vi "ANdroid_info_pusher.vi"(10 "IndexerIn":i32) -> (2 "indexout":i32, 3 "spreadsheet string":string)   [LabVIEW 2015]
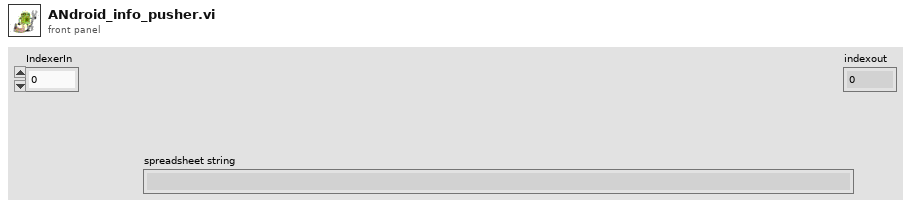
[diagram p1: front panel]
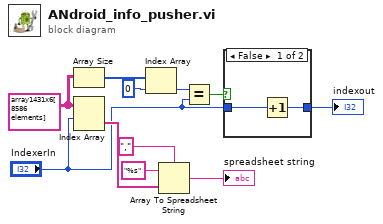
[diagram p0: block diagram]
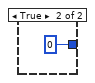
[diagram p2: hidden frame]
diagram:
  w2 = string[][] array1431x6[8586 elements] ("subarray 2")
  n1 = Array Size(array=w2) -> (size(s)=w7:i32[])
  n2 = Index Array(array=w2, index (row)="IndexerIn") -> (element=w9:string[])  [unwired: 1 in]
  n3 = Index Array(array=w7, index=0) -> (element=w5:i32)
  n4 = Array To Spreadsheet String(delimiter (Tab)=",", array=w9, 3:"%s" ("format string")) -> (spreadsheet string=→"spreadsheet string":string)
  n5 = Equal?(x=w5, y="IndexerIn") -> (x = y?=w4:bool)
  n6 = case shown="False" w4 {
    tunnel: [w13 0] -> w8
    tunnel: "IndexerIn" -> [w12 _]
    frame False {
      n7 = Increment(x=w12) -> (x+1=w13:i32)
    }
    frame True {
    }
  }
  "indexout" <- w8
